vi "Get Image Difference.vi"(0 "Acquisition Image In":T1, 5 "Channel Array In":dbl[](array[numeric]), 7 "Image Difference Buffers":T2, 11 "error in (no error)":errorcluster) -> (4 "Acquisition Image Out":T1, 6 "Channel Array Out":dbl[](array[numeric]), 15 "error out":errorcluster)   [LabVIEW 2012, in "Image Difference Custom Device.lvlib"]
uses:
  Image Difference Custom Device.lvlib
  <vilib>/vision/Image Controls.llb/IMAQ Image.ctl
  TypeDefs/Image Difference Info.ctl
  <vilib>/vision/NI_Vision_Development_Module.lvlib
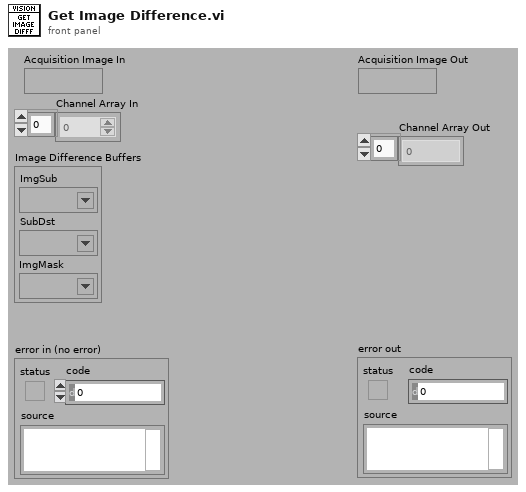
[diagram p1: front panel]
types:
  T1 = typedef "IMAQ Image.ctl" = refnum<image>
  T2 = typedef "Image Difference Custom Device.lvlib/Image Difference Info.ctl" = cluster{"ImgSub":T1, "SubDst":T1, "ImgMask":T1}
  T3 = cluster{"histogram":u32[], "Minimal Value":sgl, "Maximal Value":sgl, "Starting Value":sgl, "Interval Width":sgl, "Mean Value":sgl, "Standard  Variation":sgl, "Area (pixels)":i32}
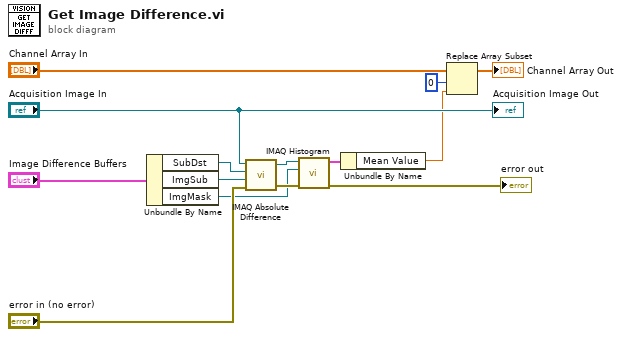
[diagram p0: block diagram]
diagram:
  n1 = Unbundle By Name("Image Difference Buffers") -> ("SubDst"=w10:T1, "ImgSub"=w9:T1, "ImgMask"=w1:T1)
  n2 = call "IMAQ Absolute Difference"("Image Src A"="Acquisition Image In", "Image Dst"=w10, "Image Src B"=w9, "error in (no error)"="error in (no error)") -> ("Image Dst Out"=w4:T1, "error out"=w5:errorcluster)  [unwired: 3 in]
  "error out" <- w5
  n3 = call "IMAQ Histogram"("error in (no error)"=w5, "Image Mask"=w1, "Image"=w4) -> ("Histogram Report"=w3:T3)  [unwired: 7 in, 1 out]
  n4 = Unbundle By Name(w3) -> ("Mean Value"=w2:sgl)
  n5 = Replace Array Subset(array="Channel Array In", new element=w2, index=0) -> (→"Channel Array Out":dbl[])
  "Acquisition Image Out" <- "Acquisition Image In"
